vi "GBF1.vi"(2 "Waveform":enum16{"SIN"}(ring), 3 "Fréquence":dbl(knob) scale=0.0..10000.0, 4 "Amplitude":dbl(knob) scale=0.0..10.0, 5 "Ressource GPIB VISA":refnum<visa-resource-name>="GPIB0::2::INSTR") -> ()   [LabVIEW 2024]
panel:
  out "Chaîne":string
  out "Données brutes":string
  out "Adresse GPIB":string
  out "?":dbl
  out "?":dbl
  # "VI GBF HAMEGH 8130"
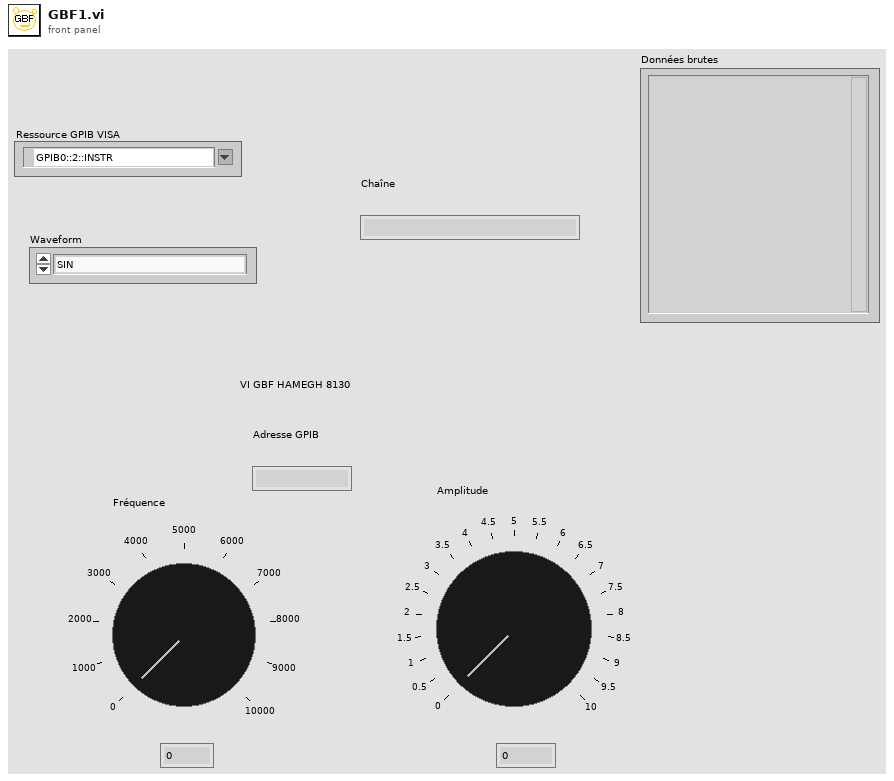
[diagram p1: front panel]
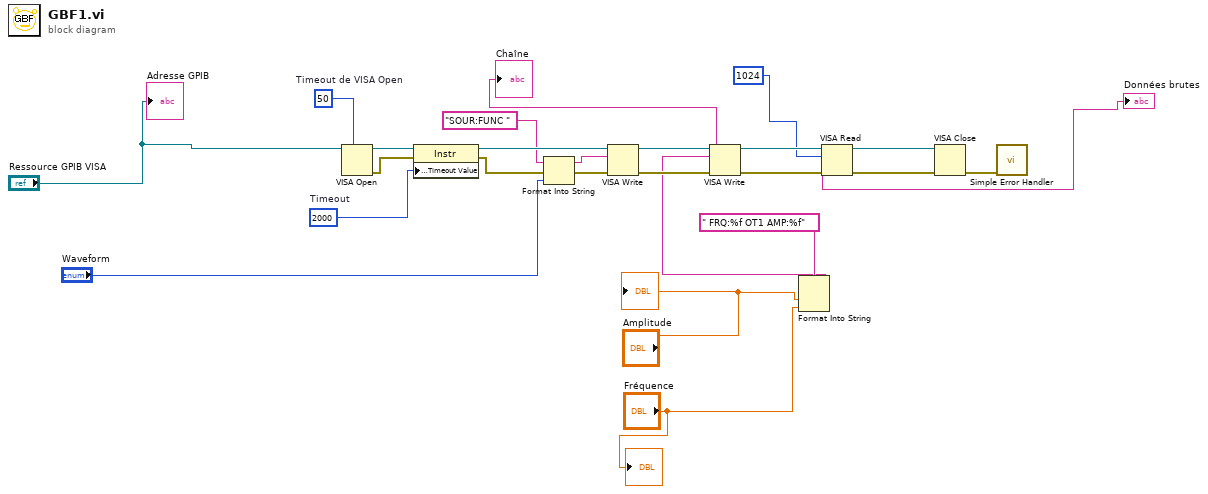
[diagram p0: block diagram]
diagram:
  w19 = u32 2000  # Timeout
  w20 = u32 50  # Timeout de VISA Open
  n1 = VISA Open(timeout (0)=w20, VISA resource name="Ressource GPIB VISA") -> (VISA resource name=w18:refnum<visa-resource-name>, error out=w17:errorcluster)  [unwired: 3 in]
  n2 = property class="Instr"(reference=w18, error in=w17, "General Settings:Timeout Value"=w19) -> (reference out=w15:refnum<visa-resource-name>, error out=w12:errorcluster)
  n3 = Format Into String(initial string="SOUR:FUNC " ("string"), error in=w12, "Waveform") -> (resulting string=w9:string, error out=w11:errorcluster)  [unwired: 1 in]
  n4 = VISA Write(VISA resource name=w15, write buffer=w9, error in (no error)=w11) -> (VISA resource name out=w14:refnum<visa-resource-name>, error out=w13:errorcluster)  [unwired: 1 out]
  n5 = Format Into String(format string=" FRQ:%f OT1 AMP:%f" ("chaîne de format"), "Amplitude", "Fréquence") -> (resulting string=w2:string)  [unwired: 2 in, 1 out]
  "Chaîne" <- w2
  n6 = VISA Write(VISA resource name=w14, write buffer=w2, error in (no error)=w13) -> (VISA resource name out=w24:refnum<visa-resource-name>, error out=w22:errorcluster)  [unwired: 1 out]
  n7 = VISA Read(VISA resource name=w24, byte count=1024, error in (no error)=w22) -> (VISA resource name out=w23:refnum<visa-resource-name>, read buffer=→"Données brutes":string, error out=w21:errorcluster)  [unwired: 1 out]
  n8 = VISA Close(VISA resource name=w23, error in (no error)=w21) -> (error out=w16:errorcluster)
  n9 = call <vilib>:"Simple Error Handler.vi"("error in (no error)"=w16) -> ()  [unwired: 4 in, 5 out]
  "?" <- "Fréquence"
  "?" <- "Amplitude"
  "Adresse GPIB" <- "Ressource GPIB VISA"
